vi "my_DAQmx_quadencoder.vi"() -> ()   [LabVIEW 2014]
doc: "I. Description:\nThis example demonstrates how to measure angular position using a quadrature encoder on a Counter Input Channel. The Decoding Type, Pulses Per Revolution, Z Index Enable, Z Index Phase, and Z Index Value are all configurable.\n\nPosition is measured on the counter's default A, B, and Z input terminals (refer to section IV, I/O Connections Overview, for more information).\n\nII. Instructions for Running:\n1. Select the Physical Channel which corresponds to the counter you want to measure position on the DAQ device.\n2. Enter the Decoding Type, Pulses Per Revolution, Z Index Enable, Z Index Phase, and Z Index Value to specify how you want the counter to measure position. \n\nIII. Block Diagram Steps:\n1. Create a Counter Input channel to Angular Encoder. The Decoding Type, Pulses Per Revolution, Z Index Enable, Z Index Phase, Z Index Value parameters are used to determine how the counter should measure position. \n2. Call the Start VI to arm the counter and begin measuring. The counter will be preloaded with the Initial Angle.\n3. The counter will be continually polled until the Stop button is pressed on the front panel.\n4. Call the Clear Task VI to clear the Task.\n5. Use the popup dialog box to display an error if any.\n\nIV. I/O Connections Overview:\nThe counter will measure position on the A, B, and Z Input Terminals of the counter specified in the Physical Channel I/O control.\n\nPosition measurement only works with TIO counters. \n\nFor more information on the default counter input and output terminals for your device, open the NI-DAQmx Help, and refer to Counter Signal Connections found under the Device Considerations book in the table of contents."
uses:
  statecontrol.ctl
  <vilib>/Utility/error.llb/DialogType.ctl
  <vilib>/LabVIEW Interface for Arduino/Type Defs/Board Type.ctl
  <vilib>/LabVIEW Interface for Arduino/Type Defs/Connection Type.ctl
  <vilib>/LabVIEW Interface for Arduino/Type Defs/Pin Mode.ctl
  <vilib>/LabVIEW Interface for Arduino/Type Defs/Arduino Resource.ctl
  <vilib>/DAQmx/read.llb/DAQmx Read (Counter 1D DBL 1Chan NSamp).vi
  <vilib>/DAQmx/create/channels.llb/DAQmx Create Channel (CI-Position-Linear Encoder).vi
  <vilib>/DAQmx/configure/task.llb/DAQmx Configure Logging (TDMS).vi
  <vilib>/DAQmx/configure/timing.llb/DAQmx Timing (Sample Clock).vi
  <vilib>/DAQmx/miscellaneous.llb/DAQmx Fill In Error Info.vi
  <resource>/objmgr/daqmx.rc
  <vilib>/LabVIEW Interface for Arduino/LabVIEW Interface for Arduino.lvlib
panel:
  out "Is the button pressed?":bool
  out "Superlight State":T1
  out "cooldown status":bool
  out "Cooldown Time Left":u32 format="%<%M:%S>t"
  out "superlight status":bool
  out "Cooldown Start Time":u32
  in  "stop":bool
  out "Superlight On Start Time":u32
  out "Tab Control":enum32{" On", "Off", "CoolDown"}(tab)
  in  "Off":bool
  in  "Frequency":dbl=5000.0 format="%#_13g"
  out "Waveform Graph":cluster{dbl, dbl, "data":dbl[]}(graph)
  out "Actual Frequency":dbl
  out "Output":dbl[](array[numeric])
  in  "number of samples":i32=1000
  in  "file path":path=path "C:/Users/Public/Documents/National Instruments/VIs/disp_history.tdms"
  in  "Decoding Type":i32(ring)=10092 items=["X1"=10090, "X2"=10091, "X4"=10092, "Two Pulse Counting"=10313]
  in  "Z Index Phase":i32(ring)=10040 items=["A High B High"=10040, "A High B Low"=10041, "A Low B High"=10042, "A Low B Low"=10043]
  in  "Z Index Value":dbl
  in  "Z Index Enable":bool
  in  "Counter(s)":tag="cDAQ1Mod1/ctr1"
  # "For instructions, select Help>>Show Context Help"
  # "Channel Parameters"
  # "Don't use ctr0, it's the clock source"
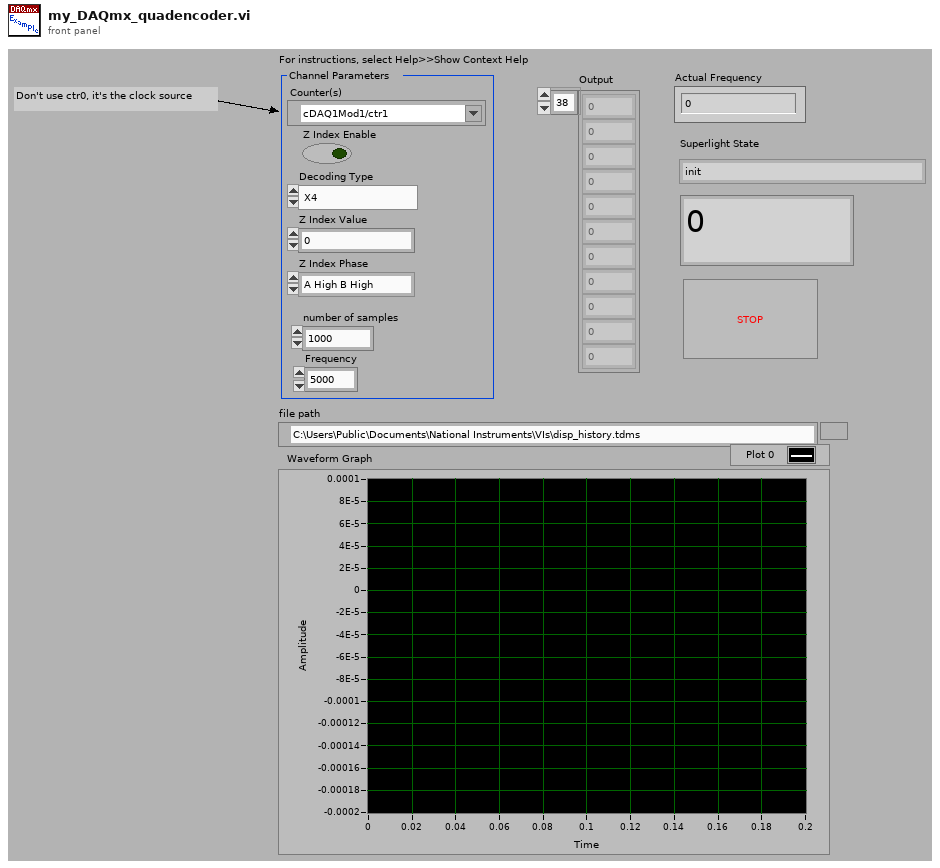
[diagram p1: front panel]
types:
  T1 = typedef "statecontrol.ctl" = enum16{"init", "waiting for trigger", "superlight on", "cooldown", "closing", "shutdown"}
  T2 = typedef "DialogType.ctl" = u16
  T3 = typedef "LabVIEW Interface for Arduino.lvlib/Pin Mode.ctl" = enum8{"Input", "Output"}
  T4 = typedef "LabVIEW Interface for Arduino.lvlib/Connection Type.ctl" = enum8{"USB / Serial", "XBEE", "BlueSmirf (Bluetooth)"}
  T5 = typedef "LabVIEW Interface for Arduino.lvlib/Board Type.ctl" = enum16{"Uno", "Dimuelanove w/Atmega 328", "Mega 2560"}
  T6 = typedef "LabVIEW Interface for Arduino.lvlib/Arduino Resource.ctl" = cluster{"VISA resource":refnum<visa-resource-name>, "Board Type":T5, "Connection Type":enum8{"USB / Serial"}, "Bytes Per Packet (15)":u8}
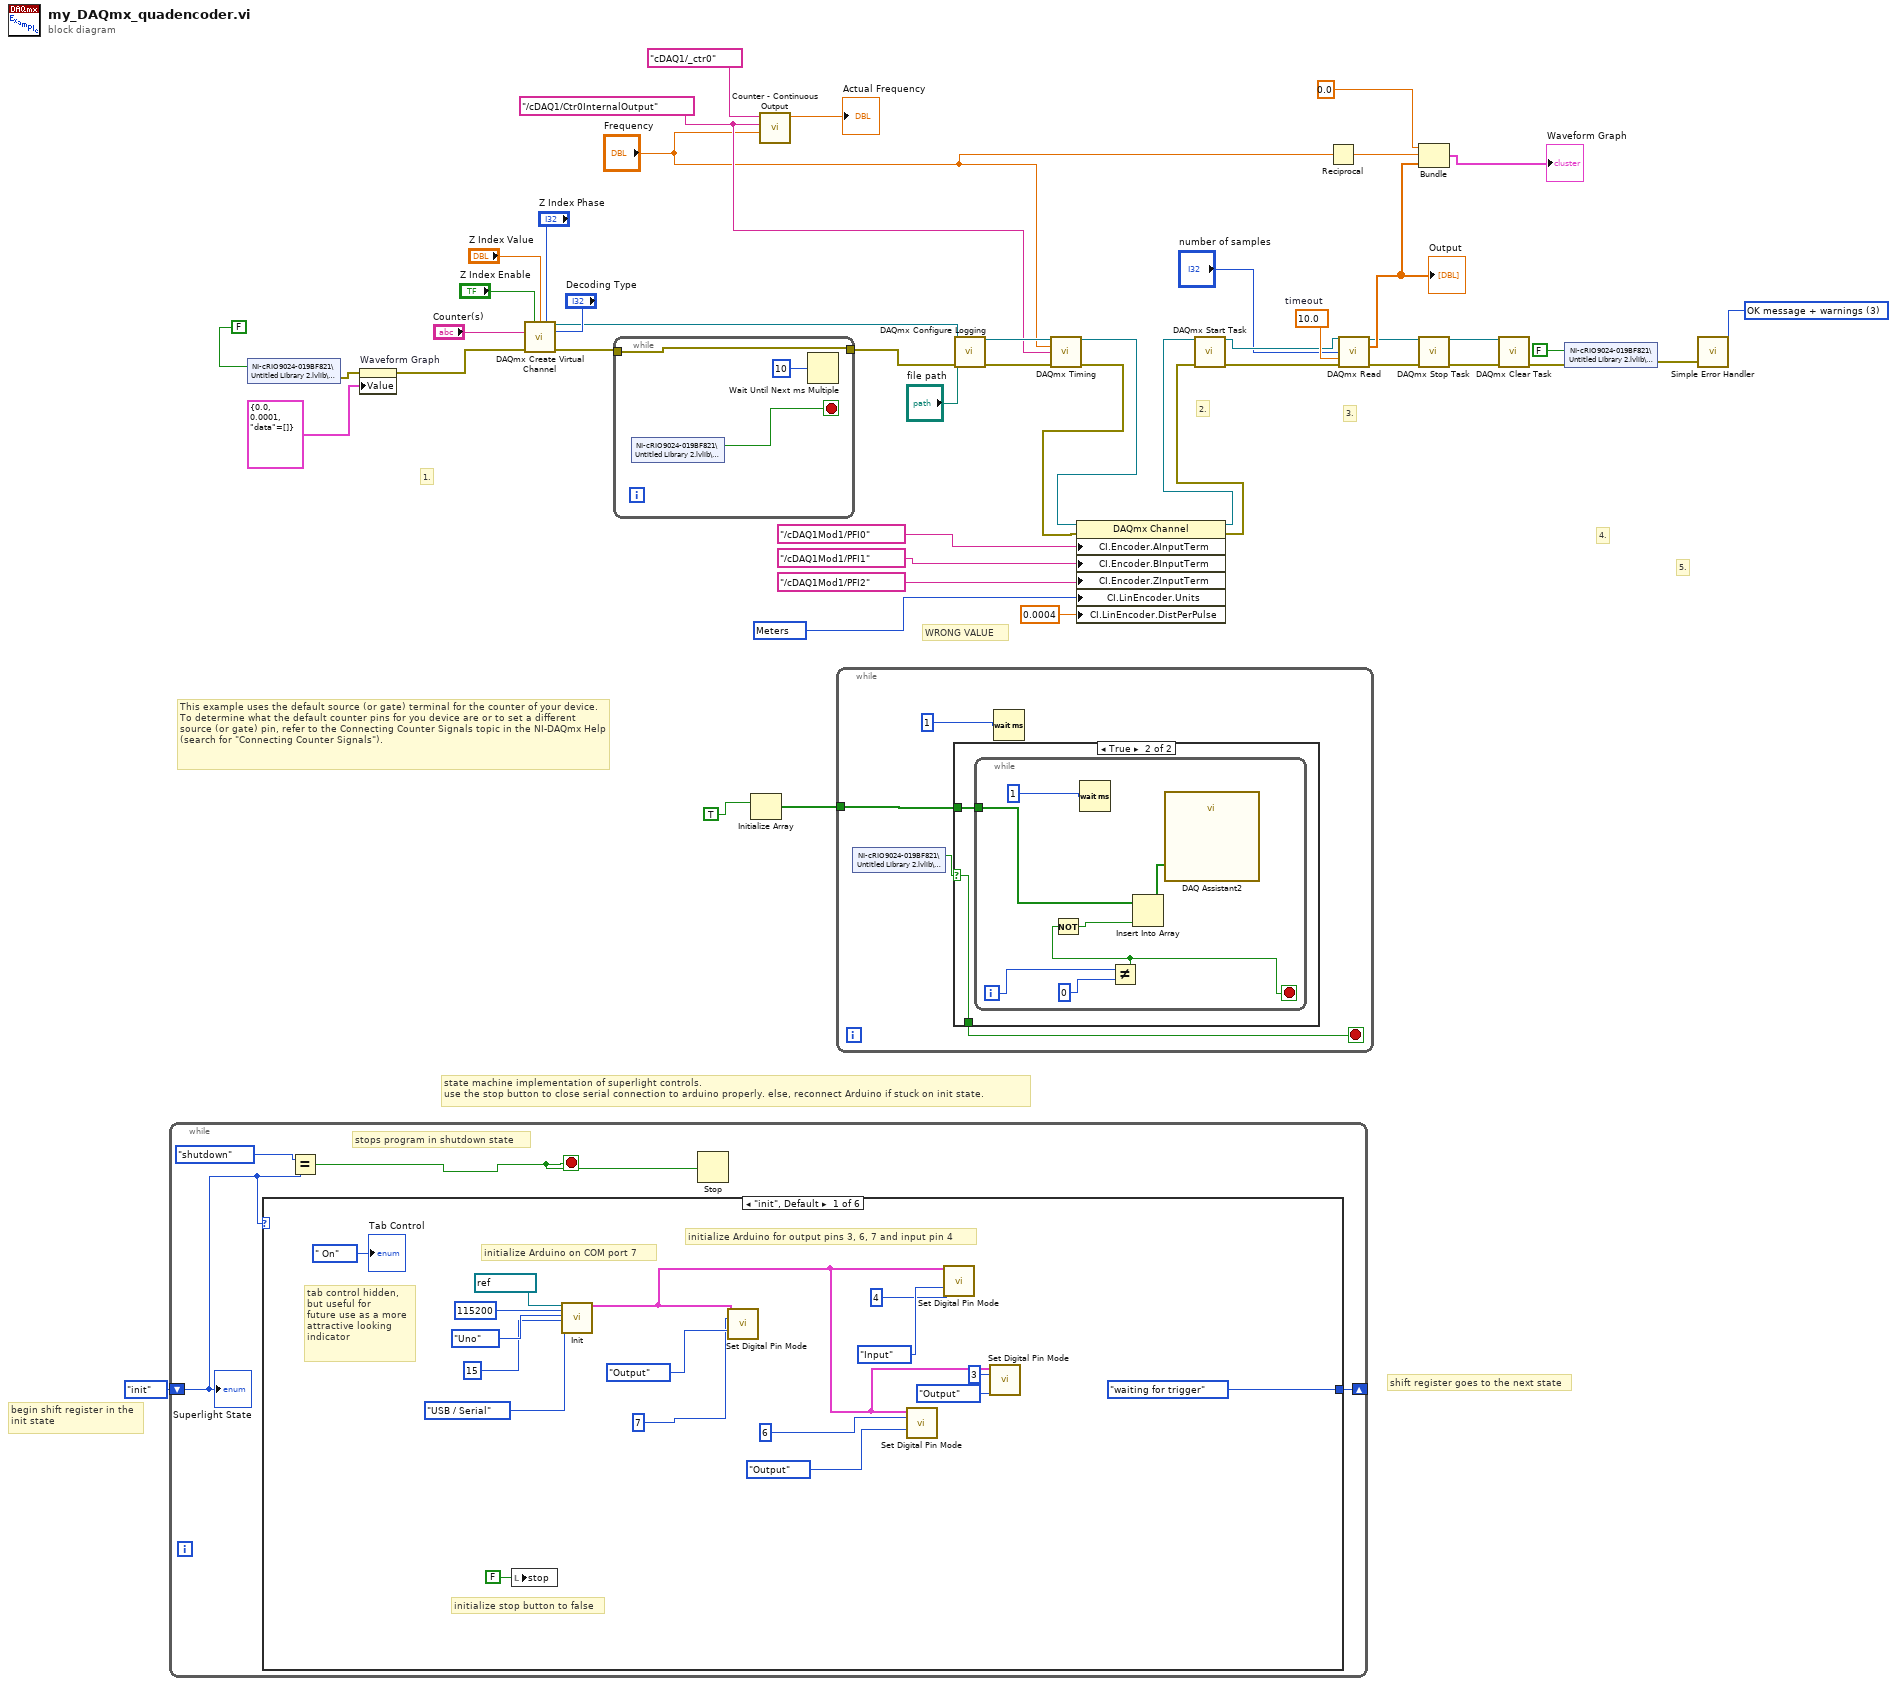
[diagram p0: block diagram]
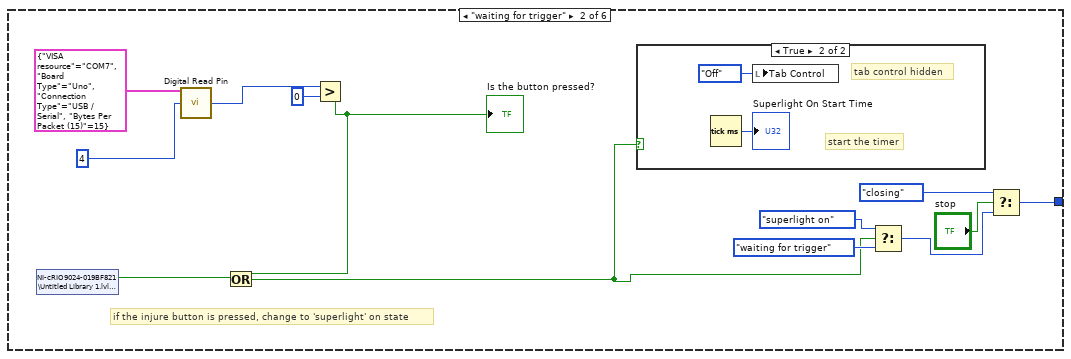
[diagram p2: hidden frame]
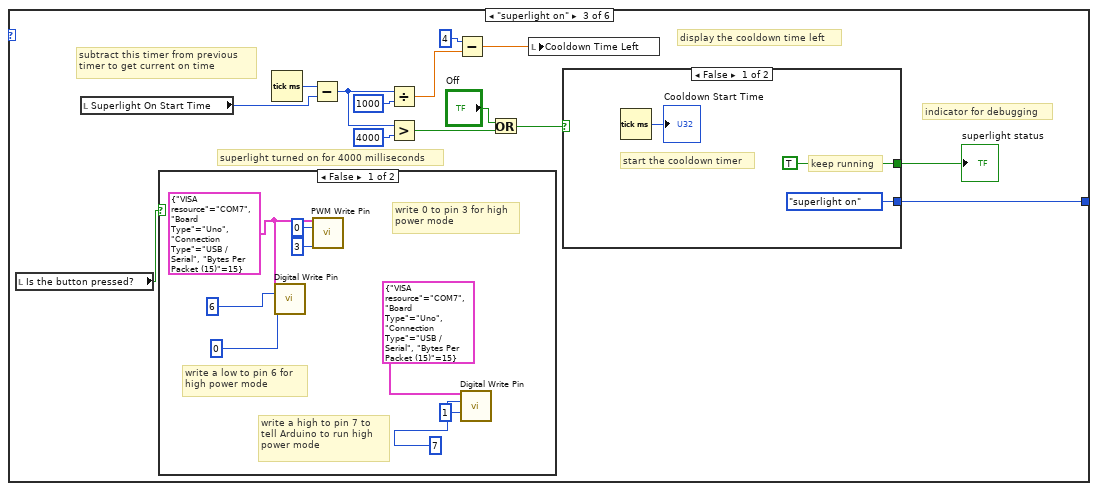
[diagram p4: hidden frame]
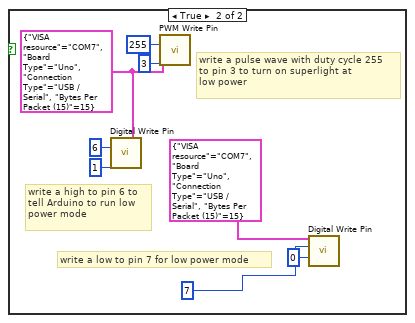
[diagram p5: hidden frame]
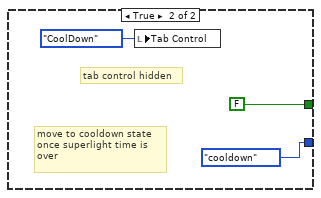
[diagram p6: hidden frame]
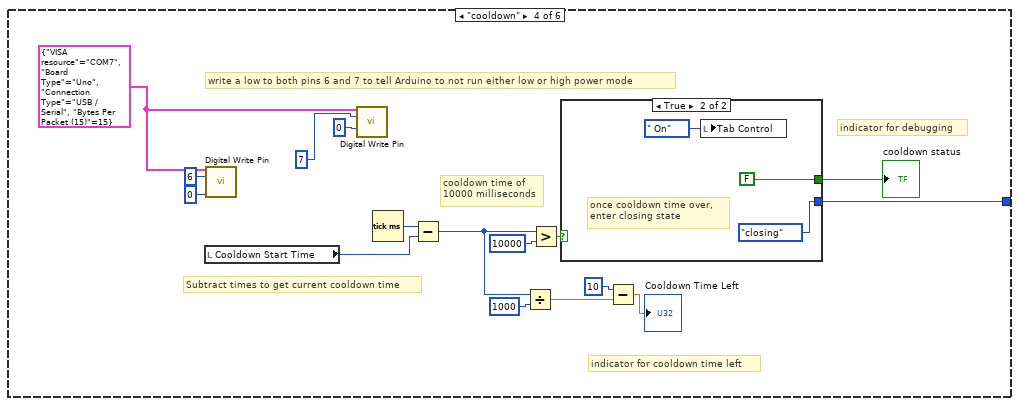
[diagram p7: hidden frame]
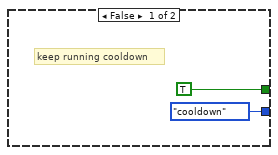
[diagram p8: hidden frame]
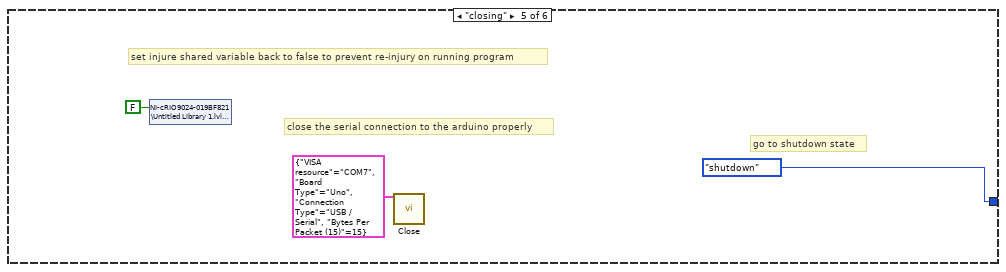
[diagram p9: hidden frame]
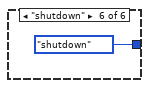
[diagram p10: hidden frame]
diagram:
  w32 = tag "/cDAQ1/Ctr0InternalOutput" ("Output Terminal")
  w34 = 10219 items=["Meters"=10219, "Inches"=10379, "Ticks"=10304, "From Custom Scale"=10065] ("CI.LinEncoder.Units")
  w39 = 10.0  # timeout
  w46 = T2 3 items=["no dialog", "OK message", "continue or stop message", "OK message + warnings", "continue/stop + warnings"] ("type of dialog (OK msg:1)")
  # "state machine implementation of superlight controls. \nuse the stop button to close serial connection to arduino properly. else, reconnect Arduino if stuck on init state."
  # "shift register goes to the next state"
  # "begin shift register in the\ninit state"
  # "WRONG VALUE"
  # "3."
  # "This example uses the default source (or gate) terminal for the counter of your device.  To determine what the default counter pins for you device are or to set a different source (or gate) pin, refer to the Connecting Counter Signals topic in the NI-DAQmx Help (search for \"Connecting Counter Signals\")."
  # "5."
  # "4."
  # "2."
  # "1."
  n1 = while {
    shift-right: [w51] -> _
    shift-left: statecontrol."init" ("state") -> [w49]
    stop <- w48 stop-if-true
    # "stops program in shutdown state"
    n2 = case shown="\"init\", Default" w49 {
      tunnel: [statecontrol."waiting for trigger" ("state") w76 w94 w131 statecontrol."shutdown" ("state") statecontrol."shutdown" ("state")] -> w51
      frame "init", Default {
        # "tab control hidden,\nbut useful for \nfuture use as a more\nattractive looking\nindicator"
        # "initialize stop button to false"
        # "initialize Arduino on COM port 7"
        # "initialize Arduino for output pins 3, 6, 7 and input pin 4"
        n3 = local write "stop"(FALSE ("stop")) -> ()
        n4 = call <vilib>:"Init.vi"("VISA resource"=refnum<visa-resource-name> "COM7", "Baud Rate (115200)"=u32 115200, "Board Type (Uno)"=Board_Type."Uno", "Bytes Per Packet (15)"=u32 15, "Connection Type (USB/Serial)"=Connection_Type."USB / Serial") -> ("Arduino Resource"=w54:T6)  [unwired: 13 in, 1 out]
        n5 = call <vilib>:"Set Digital Pin Mode.vi"("Arduino Resource"=w54, "Digital I/O Pin"=u8 7, "Pin Mode (Input)"=Pin_Mode."Output") -> ()  [unwired: 11 in, 2 out]
        n6 = call <vilib>:"Set Digital Pin Mode.vi"("Arduino Resource"=w54, "Digital I/O Pin"=u8 6, "Pin Mode (Input)"=Pin_Mode."Output") -> ()  [unwired: 11 in, 2 out]
        n7 = call <vilib>:"Set Digital Pin Mode.vi"("Arduino Resource"=w54, "Digital I/O Pin"=u8 4, "Pin Mode (Input)"=Pin_Mode."Input") -> ()  [unwired: 11 in, 2 out]
        n8 = call <vilib>:"Set Digital Pin Mode.vi"("Arduino Resource"=w54, "Digital I/O Pin"=u8 3, "Pin Mode (Input)"=Pin_Mode."Output") -> ()  [unwired: 11 in, 2 out]
        "Tab Control" <- enum32{" On", "Off", "CoolDown"}." On" ("Tab Control")
      }
      frame "waiting for trigger" {
        # "if the injure button is pressed, change to 'superlight' on state"
        n9 = shared-variable "NI-cRIO9024-019BF821\\Untitled Library 1.lvlib\\INJURE"() -> (w71:bool)  [unwired: 1 in, 1 out]
        n10 = call <vilib>:"Digital Read Pin.vi"("Arduino Resource"=T6 {"VISA resource"="COM7", "Board Type"=enum."Uno", "Connection Type"=enum."USB / Serial", "Bytes Per Packet (15)"=15}, "Digital I/O Pin (0)"=u8 4) -> ("Value"=w73:u8)  [unwired: 11 in, 2 out]
        n11 = Greater?(x=w73, y=u8 0) -> (0:w70:bool)
        "Is the button pressed?" <- w70
        n12 = Or(x=w70, y=w71) -> (x .or. y?=w69:bool)
        n13 = case shown="True" w69 {
          frame False {
          }
          frame True {
            # "start the timer"
            # "tab control hidden"
            n14 = Tick Count (ms)() -> (millisecond timer value=→"Superlight On Start Time":u32)
            n15 = local write "Tab Control"(enum32{" On", "Off", "CoolDown"}."Off" ("Tab Control")) -> ()
          }
        }
        n16 = Select(t=statecontrol."superlight on" ("state"), s=w69, f=statecontrol."waiting for trigger" ("state")) -> (s? t:f=w77:T1)
        n17 = Select(t=statecontrol."closing" ("state"), s="stop", f=w77) -> (s? t:f=w76:T1)
      }
      frame "superlight on" {
        # "indicator for debugging"
        # "superlight turned on for 4000 milliseconds"
        # "display the cooldown time left"
        # "subtract this timer from previous \ntimer to get current on time"
        n18 = local read "Is the button pressed?"() -> (w85:bool)
        n19 = local read "Superlight On Start Time"() -> (w97:u32)
        n20 = case shown="False" w85 {
          frame False {
            w101 = T6 {"VISA resource"="COM7", "Board Type"=enum."Uno", "Connection Type"=enum."USB / Serial", "Bytes Per Packet (15)"=15} ("Arduino Resource")
            # "write 0 to pin 3 for high\npower mode"
            # "write a high to pin 7 to \ntell Arduino to run high \npower mode"
            # "write a low to pin 6 for \nhigh power mode"
            n21 = call <vilib>:"Digital Write Pin.vi"("Arduino Resource"=w101, "Digital I/O Pin (0)"=u8 6, "Value (0)"=u8 0) -> ()  [unwired: 11 in, 2 out]
            n22 = call <vilib>:"PWM Write Pin.vi"("Arduino Resource"=w101, "Duty Cycle (0 - 255)"=u8 0, "PWM Pin (3)"=u8 3) -> ()  [unwired: 11 in, 2 out]
            n23 = call <vilib>:"Digital Write Pin.vi"("Arduino Resource"=T6 {"VISA resource"="COM7", "Board Type"=enum."Uno", "Connection Type"=enum."USB / Serial", "Bytes Per Packet (15)"=15}, "Digital I/O Pin (0)"=u8 7, "Value (0)"=u8 1) -> ()  [unwired: 11 in, 2 out]
          }
          frame True {
            w111 = T6 {"VISA resource"="COM7", "Board Type"=enum."Uno", "Connection Type"=enum."USB / Serial", "Bytes Per Packet (15)"=15} ("Arduino Resource")
            # "write a low to pin 7 for low power mode"
            # "write a high to pin 6 to \ntell Arduino to run low \npower mode"
            # "write a pulse wave with duty cycle 255\nto pin 3 to turn on superlight at\nlow power"
            n24 = call <vilib>:"Digital Write Pin.vi"("Arduino Resource"=w111, "Digital I/O Pin (0)"=u8 6, "Value (0)"=u8 1) -> ()  [unwired: 11 in, 2 out]
            n25 = call <vilib>:"PWM Write Pin.vi"("Arduino Resource"=w111, "Duty Cycle (0 - 255)"=u8 255, "PWM Pin (3)"=u8 3) -> ()  [unwired: 11 in, 2 out]
            n26 = call <vilib>:"Digital Write Pin.vi"("Arduino Resource"=T6 {"VISA resource"="COM7", "Board Type"=enum."Uno", "Connection Type"=enum."USB / Serial", "Bytes Per Packet (15)"=15}, "Digital I/O Pin (0)"=u8 7, "Value (0)"=u8 0) -> ()  [unwired: 11 in, 2 out]
          }
        }
        n27 = Tick Count (ms)() -> (millisecond timer value=w96:u32)
        n28 = Subtract(x=w96, y=w97) -> (x-y=w84:u32)
        n29 = Divide(x=w84, y=u32 1000) -> (x/y=w91:dbl)
        n30 = Greater?(x=w84, y=u32 4000) -> (0:w88:bool)
        n31 = Subtract(x=u32 4, y=w91) -> (x-y=w86:dbl)
        n32 = Or(x="Off", y=w88) -> (x .or. y?=w87:bool)
        n33 = local write "Cooldown Time Left"(w86) -> ()
        n34 = case shown="False" w87 {
          tunnel: [TRUE FALSE] -> w95
          tunnel: [statecontrol."superlight on" ("state") statecontrol."cooldown" ("state")] -> w94
          frame False {
            # "start the cooldown timer"
            # "keep running"
            n35 = Tick Count (ms)() -> (millisecond timer value=→"Cooldown Start Time":u32)
          }
          frame True {
            # "move to cooldown state\nonce superlight time is\nover"
            # "tab control hidden"
            n36 = local write "Tab Control"(enum32{" On", "Off", "CoolDown"}."CoolDown" ("Tab Control")) -> ()
          }
        }
        "superlight status" <- w95
      }
      frame "cooldown" {
        w120 = T6 {"VISA resource"="COM7", "Board Type"=enum."Uno", "Connection Type"=enum."USB / Serial", "Bytes Per Packet (15)"=15} ("Arduino Resource")
        # "Subtract times to get current cooldown time"
        # "write a low to both pins 6 and 7 to tell Arduino to not run either low or high power mode"
        # "indicator for cooldown time left"
        # "cooldown time of \n10000 milliseconds"
        # "indicator for debugging"
        n37 = local read "Cooldown Start Time"() -> (w135:u32)
        n38 = call <vilib>:"Digital Write Pin.vi"("Arduino Resource"=w120, "Digital I/O Pin (0)"=u8 6, "Value (0)"=u8 0) -> ()  [unwired: 11 in, 2 out]
        n39 = call <vilib>:"Digital Write Pin.vi"("Arduino Resource"=w120, "Digital I/O Pin (0)"=u8 7, "Value (0)"=u8 0) -> ()  [unwired: 11 in, 2 out]
        n40 = Tick Count (ms)() -> (millisecond timer value=w134:u32)
        n41 = Subtract(x=w134, y=w135) -> (x-y=w127:u32)
        n42 = Divide(x=w127, y=u32 1000) -> (x/y=w128:dbl)
        n43 = Greater?(x=w127, y=u32 10000) -> (0:w133:bool)
        n44 = case shown="True" w133 {
          tunnel: [TRUE FALSE] -> w132
          tunnel: [statecontrol."cooldown" ("state") statecontrol."closing" ("state")] -> w131
          frame False {
            # "keep running cooldown"
          }
          frame True {
            # "once cooldown time over,\nenter closing state"
            n45 = local write "Tab Control"(enum32{" On", "Off", "CoolDown"}." On" ("Tab Control")) -> ()
          }
        }
        "cooldown status" <- w132
        n46 = Subtract(x=u32 10, y=w128) -> (x-y=→"Cooldown Time Left":dbl)
      }
      frame "closing" {
        # "go to shutdown state"
        # "set injure shared variable back to false to prevent re-injury on running program"
        # "close the serial connection to the arduino properly"
        n47 = shared-variable "NI-cRIO9024-019BF821\\Untitled Library 1.lvlib\\INJURE"(FALSE ("INJURE")) -> ()  [unwired: 1 in, 1 out]
        n48 = call <vilib>:"Close.vi"("Arduino Resource"=T6 {"VISA resource"="COM7", "Board Type"=enum."Uno", "Connection Type"=enum."USB / Serial", "Bytes Per Packet (15)"=15}) -> ()  [unwired: 14 in, 1 out]
      }
      frame "shutdown" {
      }
    }
    n49 = Equal?(x=statecontrol."shutdown" ("state"), y=w49) -> (x = y?=w48:bool)
    n50 = Stop(stop? (T)=w48) -> ()
    "Superlight State" <- w49
  }
  n51 = shared-variable "NI-cRIO9024-019BF821\\Untitled Library 2.lvlib\\Variable2"(FALSE ("Variable2")) -> (error out=w22:errorcluster)  [unwired: 1 in]
  n52 = property on="Waveform Graph" class="WFGraph (strict)"(error in=w22, "Value"=cluster{dbl, dbl, "data":dbl[]} {0.0, 0.0001, "data"=[]} ("Waveform Graph")) -> (error out=w21:errorcluster)  [unwired: 1 in, 1 out]
  n53 = call-poly <vilib>:"DAQmx Create Virtual Channel.vi"("z index enable"="Z Index Enable", "z index value"="Z Index Value", "z index phase"="Z Index Phase", "counter"="Counter(s)", "decoding type"="Decoding Type", "error in"=w21) -> ("task out"=w41:refnum<k21>, "error out"=w10:errorcluster)  [unwired: 8 in]
  n54 = while {
    tunnel: w10 -> [w146]
    tunnel: [w146] -> w4
    stop <- w145 stop-if-true
    n55 = shared-variable "NI-cRIO9024-019BF821\\Untitled Library 2.lvlib\\Variable2"() -> (w145:bool)  [unwired: 1 in, 1 out]
    n56 = Wait Until Next ms Multiple(millisecond multiple=u32 10) -> ()  [unwired: 1 out]
  }
  n57 = Initialize Array(TRUE) -> (w2:bool[])  [unwired: 1 in]
  n58 = call "Counter - Continuous Output.vi"("Frequency"="Frequency", "Output Terminal"=w32, "Counter"=tag "cDAQ1/_ctr0") -> ("Actual Frequency"=→"Actual Frequency":dbl)  [unwired: 8 in]
  n59 = while {
    tunnel: w2 -> [w149]
    stop <- w150 stop-if-true
    n60 = shared-variable "NI-cRIO9024-019BF821\\Untitled Library 2.lvlib\\Variable2"() -> (w148:bool)  [unwired: 1 in, 1 out]
    n61 = case shown="True" w148 {
      selector: w148 -> [w152 w154]
      tunnel: [w152 w154] -> w150
      tunnel: w149 -> [_ w153]
      frame False {
      }
      frame True {
        n62 = while {
          tunnel: w153 -> [w158]
          i -> [w160]
          stop <- w157 stop-if-true
          n63 = Wait (ms)(milliseconds to wait=1) -> ()  [unwired: 1 out]
          n64 = Not Equal?(x=w160, y=0) -> (x != y?=w157:bool)
          n65 = Not(x=w157) -> (.not. x?=w156:bool)
          n66 = Insert Into Array(array=w158, new element=w156) -> (w155:bool[])  [unwired: 1 in]
          n67 = call "DAQ Assistant2"("data"=w155) -> ()  [unwired: 17 in, 2 out]
        }
      }
    }
    n68 = Wait (ms)(milliseconds to wait=1) -> ()  [unwired: 1 out]
  }
  n69 = call-poly <vilib>:"DAQmx Configure Logging.vi"("task/channels in"=w41, "file path"="file path", "error in"=w4) -> ("task out"=w40:refnum<k21>, "error out"=w11:errorcluster)  [unwired: 11 in]
  n70 = call-poly <vilib>:"DAQmx Timing.vi"("task/channels in"=w40, "rate"="Frequency", "source"=w32, "error in"=w11) -> ("task out"=w13:refnum<k21>, "error out"=w12:errorcluster)  [unwired: 10 in]
  n71 = property class="DAQmx Channel"(reference=w13, error in=w12, "CI.Encoder.AInputTerm"=tag "/cDAQ1Mod1/PFI0", "CI.Encoder.BInputTerm"=tag "/cDAQ1Mod1/PFI1", "CI.Encoder.ZInputTerm"=tag "/cDAQ1Mod1/PFI2", "CI.LinEncoder.Units"=w34, "CI.LinEncoder.DistPerPulse"=0.0004) -> (reference out=w15:refnum<k21>, error out=w14:errorcluster)
  n72 = call <vilib>:"DAQmx Start Task.vi"("task/channels in"=w15, "error in"=w14) -> ("task out"=w38:refnum<k21>, "error out"=w20:errorcluster)  [unwired: 12 in]
  n73 = Reciprocal(x="Frequency") -> (1/x=w28:dbl)
  n74 = call-poly <vilib>:"DAQmx Read.vi"("task/channels in"=w38, "number of samples per channel"="number of samples", "timeout"=w39, "error in"=w20) -> ("task out"=w17:refnum<k21>, "data"=w26:dbl[], "error out"=w19:errorcluster)  [unwired: 9 in]
  "Output" <- w26
  n75 = Bundle(0.0, w28, "data"=w26) -> (→"Waveform Graph":cluster{dbl, dbl, "data":dbl[]})  [unwired: 1 in]
  n76 = call <vilib>:"DAQmx Stop Task.vi"("task/channels in"=w17, "error in"=w19) -> ("task out"=w16:refnum<k21>, "error out"=w18:errorcluster)  [unwired: 12 in]
  n77 = call <vilib>:"DAQmx Clear Task.vi"("task in"=w16, "error in"=w18) -> ("error out"=w9:errorcluster)  [unwired: 13 in]
  n78 = shared-variable "NI-cRIO9024-019BF821\\Untitled Library 2.lvlib\\Variable2"(FALSE ("Variable2"), error in=w9) -> (error out=w8:errorcluster)
  n79 = call <vilib>:"Simple Error Handler.vi"("type of dialog (OK msg:1)"=w46, "error in (no error)"=w8) -> ()  [unwired: 3 in, 5 out]
